vi "Ball Intake SS Controls to Commands 2017.vi"(11 "Pilot-CoPilot Controls":T2) -> (3 "Ball Intake Commands":T1)   [LabVIEW 2016]
uses:
  Robot Control Outputs 2017.ctl
  Ball Intake Commands.ctl
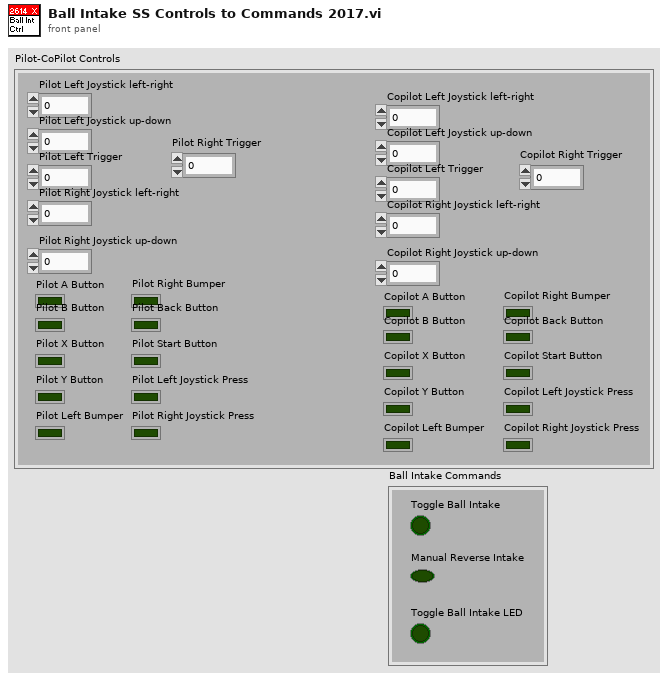
[diagram p1: front panel]
types:
  T1 = typedef "Ball Intake Commands.ctl" = cluster{"Toggle Ball Intake":bool, "Manual Reverse Intake":bool, "Toggle Ball Intake LED":bool}
  T2 = typedef "Robot Control Outputs 2017.ctl" = cluster{"Pilot Left Joystick left-right":dbl, "Pilot Left Joystick up-down":dbl, "Pilot A Button":bool, "Pilot B Button":bool, "Pilot X Button":bool, "Pilot Y Button":bool, "Pilot Left Bumper":bool, "Pilot Right Bumper":bool, "Pilot Back Button":bool, "Pilot Start Button":bool, "Pilot Left Joystick Press":bool, "Pilot Right Joystick Press":bool, "Pilot Left Trigger":dbl, "Pilot Right Joystick left-right":dbl, "Pilot Right Joystick up-down":dbl, "Pilot Right Trigger":dbl, "Copilot Left Joystick left-right":dbl, "Copilot Left Joystick up-down":dbl, "Copilot A Button":bool, "Copilot B Button":bool, "Copilot X Button":bool, "Copilot Y Button":bool, "Copilot Left Bumper":bool, "Copilot Right Bumper":bool, "Copilot Back Button":bool, "Copilot Start Button":bool, "Copilot Left Joystick Press":bool, "Copilot Right Joystick Press":bool, "Copilot Left Trigger":dbl, "Copilot Right Joystick left-right":dbl, "Copilot Right Joystick up-down":dbl, "Copilot Right Trigger":dbl}
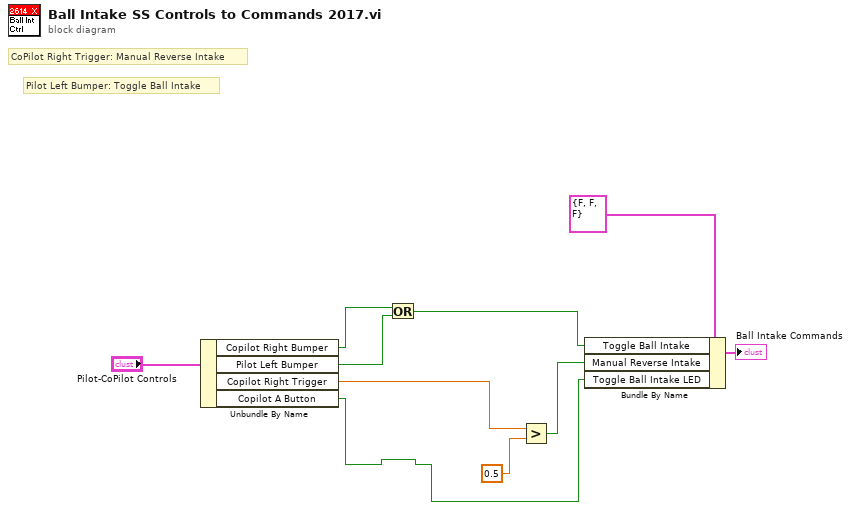
[diagram p0: block diagram]
diagram:
  # "CoPilot Right Trigger: Manual Reverse Intake"
  # "Pilot Left Bumper: Toggle Ball Intake"
  n1 = Unbundle By Name("Pilot-CoPilot Controls") -> ("Copilot Right Bumper"=w3:bool, "Pilot Left Bumper"=w4:bool, "Copilot Right Trigger"=w6:dbl, "Copilot A Button"=w1:bool)
  n2 = Or(x=w3, y=w4) -> (x .or. y?=w2:bool)
  n3 = Greater?(x=w6, y=0.5 ("x")) -> (0:w7:bool)
  n4 = Bundle By Name(cluster=T1 {"Toggle Ball Intake"=FALSE, "Manual Reverse Intake"=FALSE, "Toggle Ball Intake LED"=FALSE} ("Ball Intake Commands"), "Toggle Ball Intake"=w2, "Manual Reverse Intake"=w7, "Toggle Ball Intake LED"=w1) -> (→"Ball Intake Commands":T1)
